vi "Get NI-Scope Instrument Name.vi"(8 "Error In":errorcluster, 11 "Semiconductor Module Context":T1) -> (0 "Error Out":errorcluster, 1 "Channel Lists":string[](array[string]), 2 "Instrument Names":string[](array[string]), 3 "Semiconductor Module Context Out":T1)   [LabVIEW 2013]
uses:
  <vilib>/NI_TestStand_SemiconductorModule/NI_TestStand_Semiconductor_Module.lvlibp/PinMap/General/SemiconductorModuleContext.ctl
  <vilib>/NI_TestStand_SemiconductorModule/NI_TestStand_Semiconductor_Module.lvlibp
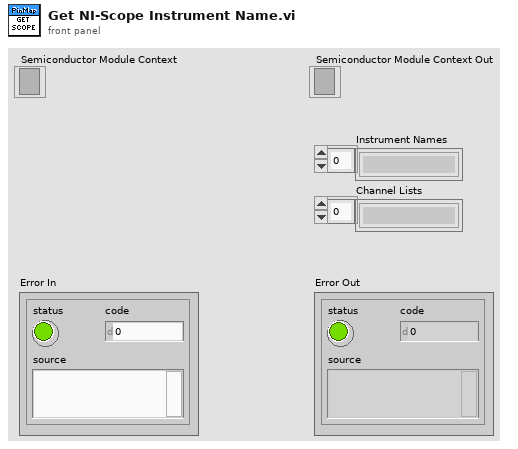
[diagram p1: front panel]
types:
  T1 = typedef "NI_TestStand_Semiconductor_Module.lvlibp/SemiconductorModuleContext.ctl" = refnum<k7>
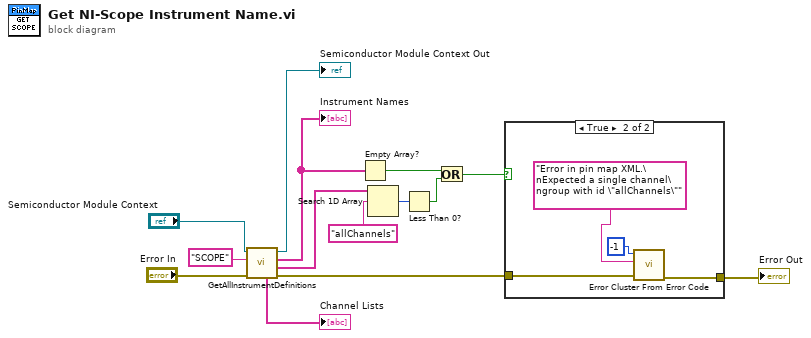
[diagram p0: block diagram]
diagram:
  n1 = call <vilib>:"GetAllInstrumentDefinitions.vi"("error in (no error)"="Error In", "Instrument Type Id"="SCOPE", "Semiconductor Module Context"="Semiconductor Module Context") -> ("error out"=w3:errorcluster, "Channel Group Ids"=w12:string[], "Instrument Names"=w11:string[], "Semiconductor Module Context Out"=→"Semiconductor Module Context Out":T1, "Channel Lists"=→"Channel Lists":string[])  [unwired: 4 in]
  "Instrument Names" <- w11
  n2 = Empty Array?(array=w11) -> (empty?=w10:bool)
  n3 = Search 1D Array(1D array=w12, element="allChannels" ("y")) -> (index of element=w8:i32)  [unwired: 1 in]
  n4 = Less Than 0?(x=w8) -> (x < 0?=w7:bool)
  n5 = Or(x=w10, y=w7) -> (x .or. y?=w1:bool)
  n6 = case shown="True" w1 {
    tunnel: w3 -> [w15 w19]
    tunnel: [w15 w16] -> w2
    frame False {
    }
    frame True {
      n7 = call <vilib>:"Error Cluster From Error Code.vi"("error in (no error)"=w19, "error message (\"\")"="Error in pin map XML.\nExpected a single channel\ngroup with id \"allChannels\"" ("error message (\"\")"), "error code (0)"=-1) -> ("error out"=w16:errorcluster)  [unwired: 6 in]
    }
  }
  "Error Out" <- w2
